vi "主界面.vi"() -> ()   [LabVIEW 2015]
panel:
  in  "停止按钮":bool
  in  "滚动方式":enum32{"左", "暂停", "右"}(radio)
  in  "速度":u32=10
  out "?":bool[][](array[boolean])
  in  "字幕内容":string="这是主vi"
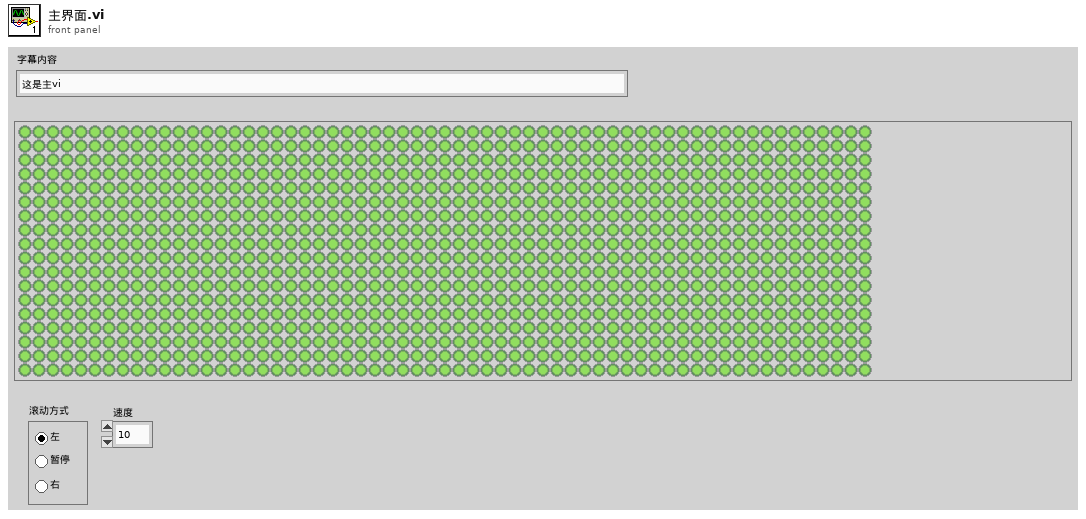
[diagram p1: front panel]
types:
  T1 = cluster{"left":i16, "top":i16, "right":i16, "bottom":i16}
  T2 = cluster{"Font Name:":string, "Size":i16, "Strikeout?":bool, "Italic?":bool, "Underline?":bool, "Outline?":bool, "Shadow?":bool, "Bold?":bool}
  T3 = enum16{"User-specified Font", "Application Font", "System Font", "Dialog Font"}
  T4 = typedef "imagedata.ctl" = cluster{"image type":i32, "image depth":i32, "image":u8[], "mask":u8[], "colors":u32[], "Rectangle":cluster{"left":i16, "top":i16, "right":i16, "bottom":i16}}
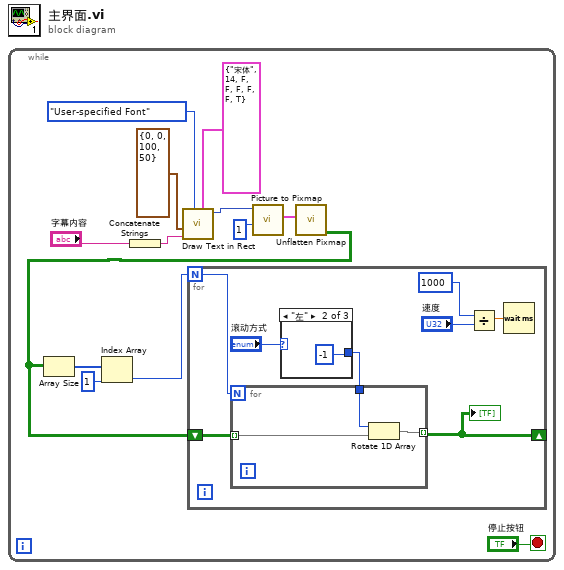
[diagram p0: block diagram]
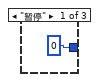
[diagram p2: hidden frame]
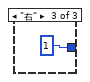
[diagram p3: hidden frame]
diagram:
  n1 = while {
    stop <- "停止按钮" stop-if-true
    n2 = Concatenate Strings("字幕内容") -> (w10:string)
    n3 = call <vilib>:"Draw Text in Rect.vi"("[user-specified font]"=T2 {"Font Name:"="宋体", "Size"=14, "Strikeout?"=FALSE, "Italic?"=FALSE, "Underline?"=FALSE, "Outline?"=FALSE, "Shadow?"=FALSE, "Bold?"=TRUE}, "desired font(Application)"=T3."User-specified Font", "text"=w10, "rect"=T1 {"left"=0, "top"=0, "right"=100, "bottom"=50}) -> ("new picture"=w13:picture)  [unwired: 7 in]
    n4 = call <vilib>:"Picture to Pixmap.vi"("depth"=1, "picture"=w13) -> ("image data"=w12:T4)  [unwired: 8 in, 1 out]
    n5 = call <vilib>:"Unflatten Pixmap.vi"("image data"=w12) -> ("1-bit pixmap"=w5:bool[][])  [unwired: 4 in, 6 out]
    n6 = Array Size(array=w5) -> (size(s)=w8:i32[])
    n7 = Index Array(array=w8, index=1 ("索引")) -> (element=w6:i32)
    n8 = for {
      N: w6 -> [w20]
      shift-right: [w19] -> _
      shift-left: w5 -> [w21]
      n9 = case shown="\"左\"" "滚动方式" {
        tunnel: [0 -1 1] -> w14
        frame "暂停" {
        }
        frame "左" {
        }
        frame "右" {
        }
      }
      n10 = for {
        N: w20 -> [_]
        tunnel: w21 -> [w27] mode=indexing
        tunnel: [w26] -> w19 mode=indexing
        tunnel: w14 -> [w25]
        n11 = Rotate 1D Array(1:w27, 2:w25) -> (0:w26:bool[])
      }
      "?" <- w19
      n12 = Divide(x=u32 1000 ("y"), y="速度") -> (x/y=w18:dbl)
      n13 = Wait (ms)(milliseconds to wait=w18) -> ()  [unwired: 1 out]
    }
  }
